vi "RADI SINHRO Peak Senzora.vi"() -> ()   [LabVIEW 2017]
uses:
  <vilib>/Waveform/WDTOps.llb/WDT Index Channel DBL.vi
panel:
  in  "Tab Control":enum32{"FRONT", "LIVE DATA", "Podesavanja"}(tab)
  in  "Brzina App":i16(slide)=1900 caption="Speed" min=500 max=1900 step=100 scale=500.0..1900.0
  out "3":bool
  out "2":bool
  out "1":bool
  out "?":dbl format="%#5_3g"
  out "TRENUTNI SIGNALI":dynamicdata(graph) caption="TRENUTNI SIGNALI !!!!"
  out "GORE":bool
  in  "Ponavljanja":i32=40
  out "ULAZ ANN":dbl[](array[numeric])
  out "Niz":dbl[](array[numeric])
  out "Matrica":dbl[][](array[numeric])
  out "BROJ":dbl
  out "SREDINA":bool
  out "DOLE":bool
  out "sum":dbl
  out "Sekvenca":dbl[](array[numeric])
  in  "Kombinacije":string(combo)="Combinations_1 - Srpski_Brojevi"
  out "Iter":i32
  out "SCORE":dbl
  in  "VREME 100mS":i16(knob)=1900 min=500 max=19000 step=100 scale=500.0..1900.0
  out "error out":errorcluster
  # "PROVERITI DA LI BROJ UDARCE"
  # "'Gore 1, Sredina 2, Dole 4, Miruje 8'"
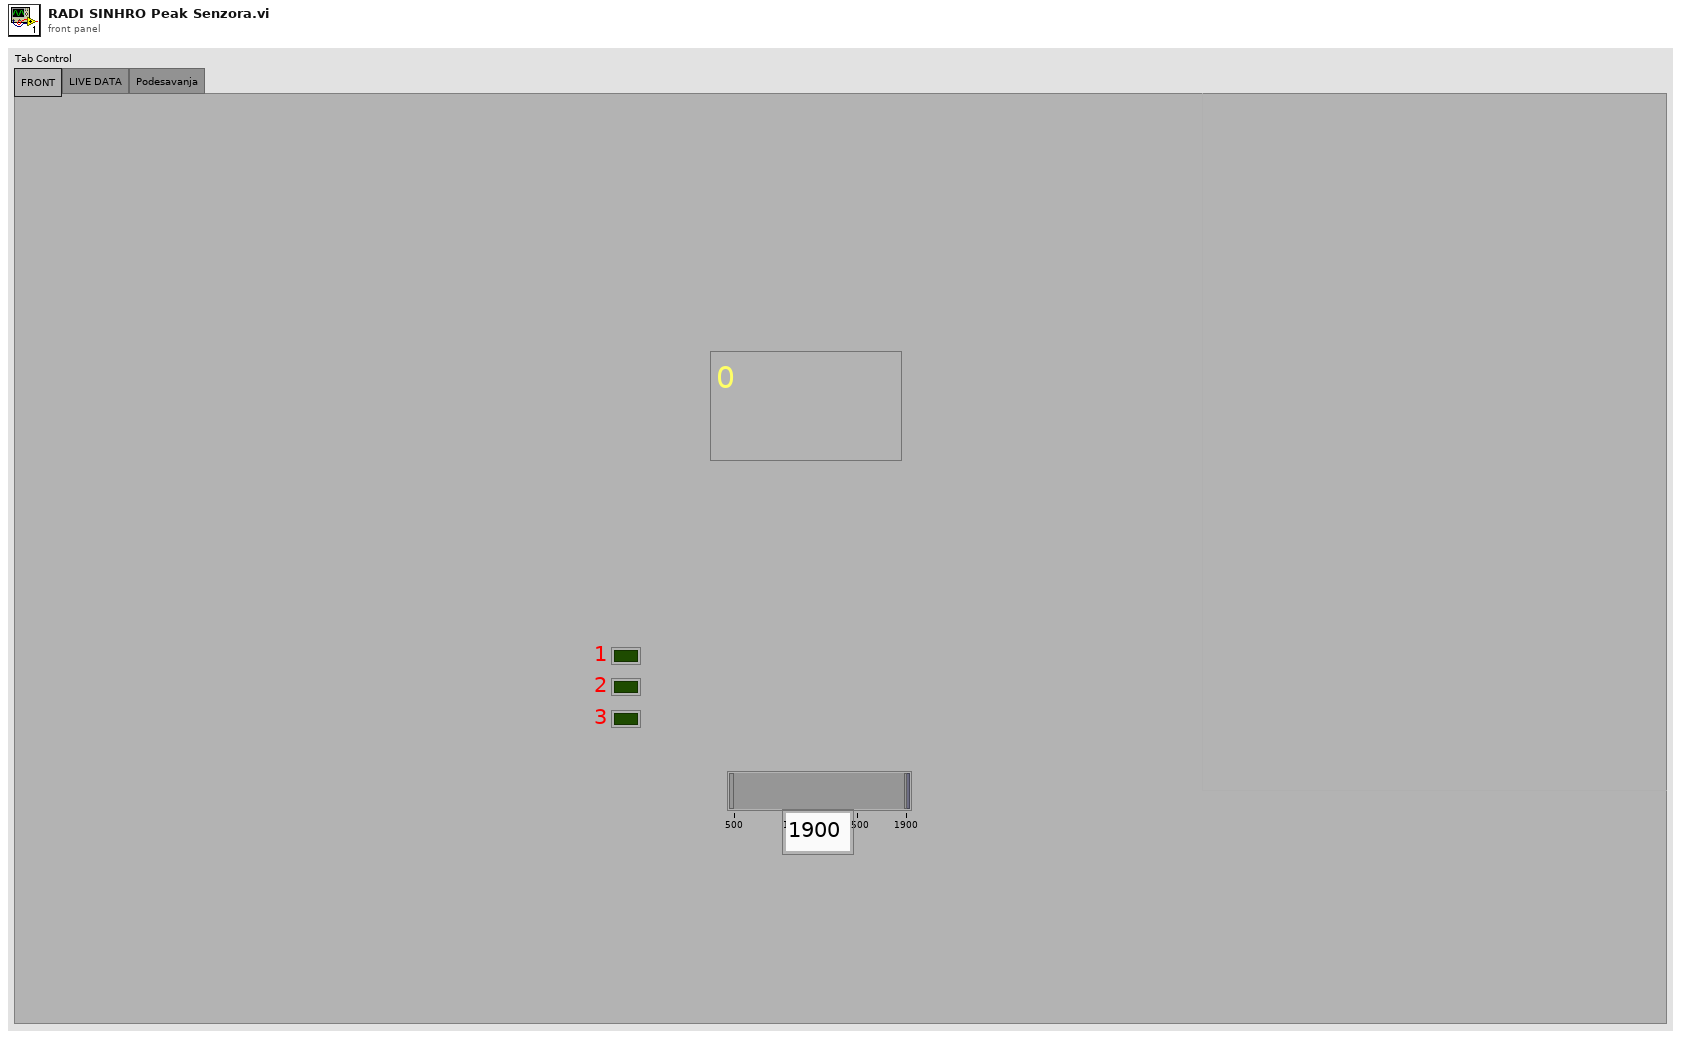
[diagram p1: front panel]
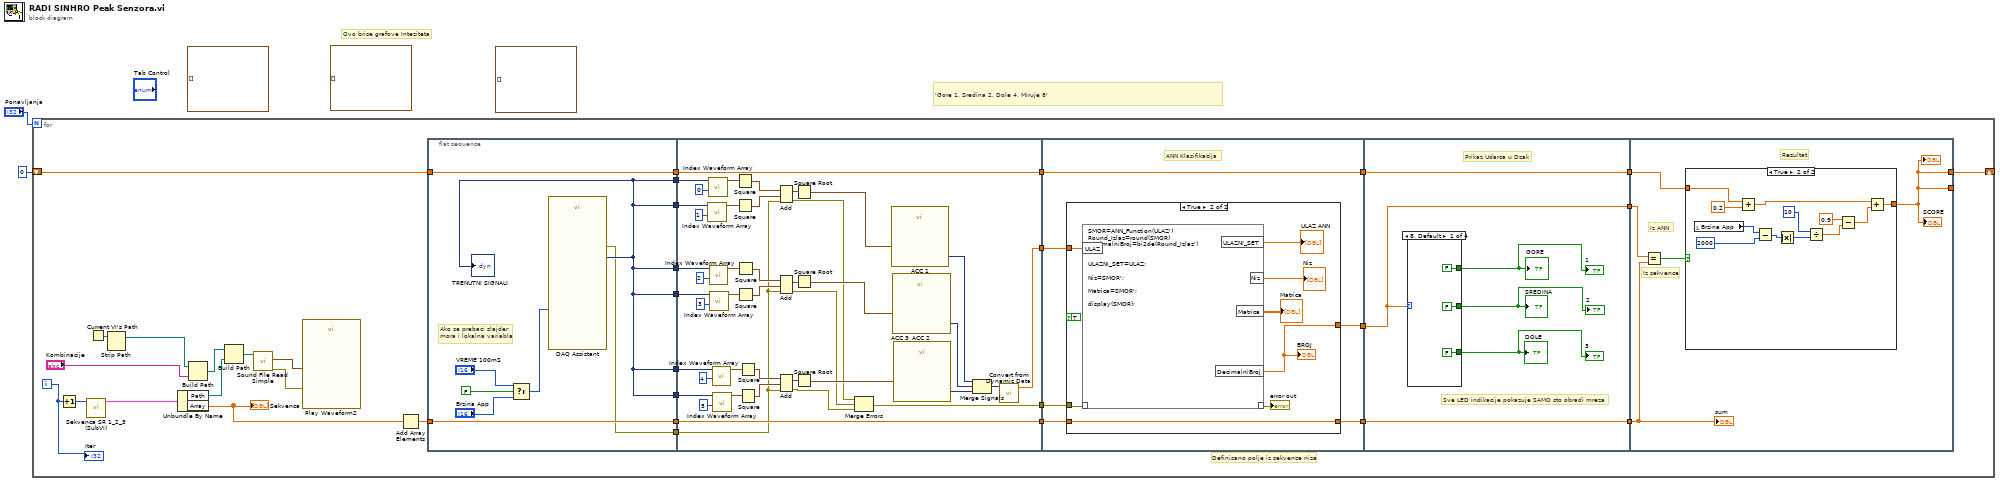
[diagram p0: block diagram]
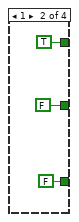
[diagram p3: hidden frame]
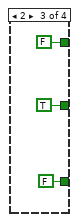
[diagram p4: hidden frame]
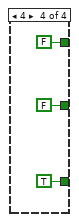
[diagram p5: hidden frame]
diagram:
  (unwired) waveform(dbl)[] [] ("History Data")
  (unwired) waveform(dbl)[] [] ("History Data")
  (unwired) waveform(dbl)[] [] ("History Data")
  # "'Gore 1, Sredina 2, Dole 4, Miruje 8'"
  # "Ovo brise grafove Inteziteta"
  n1 = for {
    N: "Ponavljanja" -> [_]
    shift-right: [w3] -> _
    shift-left: 0 -> [w25]
    i -> [w27]
    # "Definisano polje iz sekvence niza"
    n2 = Increment(x=w27) -> (x+1=w28:i32)
    n3 = call "Sekvenca SR 1_2_3 (SubVI).vi"("Ulaz"=w28) -> ("Cluster 41"=w29:cluster{"Path":path, "Array":dbl[]})  [unwired: 9 in, 1 out]
    n4 = Current VI's Path() -> (path=w35:path)
    n5 = Strip Path(path=w35) -> (stripped path=w32:path)  [unwired: 1 out]
    n6 = Unbundle By Name(w29) -> ("Path"=w30:path, "Array"=w26:dbl[])
    "Sekvenca" <- w26
    n7 = Build Path(base path=w32, name or relative path="Kombinacije") -> (appended path=w34:path)
    n8 = Build Path(base path=w34, name or relative path=w30) -> (appended path=w33:path)
    n9 = call <vilib>:"Sound File Read Simple.vi"("path"=w33) -> ("error out"=w36:errorcluster, "data"=w31:waveform(dbl)[])  [unwired: 7 in, 2 out]
    n10 = call "Play Waveform2"("Data"=w31, "error in"=w36) -> ()  [unwired: 17 in, 1 out]
    n11 = Add Array Elements(numeric array=w26) -> (sum=w19:dbl)
    n12 = flat-sequence {
      tunnel: w19 -> [w43]
      tunnel: w25 -> [w44]
      tunnel: [w44] -> w12
      tunnel: [w43] -> w11
      tunnel: [w41] -> w10
      tunnel: [w41] -> w9
      tunnel: [w41] -> w8
      tunnel: [w41] -> w7
      tunnel: [w41] -> w6
      tunnel: [w41] -> w5
      tunnel: [w37] -> w4
      tunnel: [w86] -> w16
      tunnel: [w47] -> w15
      tunnel: [w48] -> w14
      tunnel: [w85] -> w13
      tunnel: w12 -> [w86]
      tunnel: w11 -> [w85]
      tunnel: w10 -> [w59]
      tunnel: w9 -> [w57]
      tunnel: w8 -> [w55]
      tunnel: w7 -> [w53]
      tunnel: w6 -> [w51]
      tunnel: w5 -> [w49]
      tunnel: w4 -> [w45]
      tunnel: [w93] -> w21
      tunnel: [w87] -> w20
      tunnel: [w88] -> w17
      tunnel: w16 -> [w93]
      tunnel: w15 -> [w92]
      tunnel: w14 -> [w91]
      tunnel: w13 -> [w89]
      tunnel: [w105] -> w23
      tunnel: [w104] -> w22
      tunnel: w21 -> [w105]
      tunnel: w20 -> [w104]
      tunnel: [w103] -> w18
      tunnel: w17 -> [w103]
      tunnel: w23 -> [w124]
      tunnel: w22 -> [w122]
      tunnel: [w123] -> _
      tunnel: w18 -> [w121]
      tunnel: [w123] -> w3
      frame #0 {
        # "Ako se prebaci slajder\nmora i lokalna variabla"
        n13 = Select(t="VREME 100mS", s=FALSE, f="Brzina App") -> (s? t:f=w42:i16)
        n14 = call "DAQ Assistant"("number of samples"=w42) -> ("data"=w41:dynamicdata, "error out"=w37:errorcluster)  [unwired: 15 in, 2 out]
        "TRENUTNI SIGNALI" <- w41
      }
      frame #1 {
        n15 = call-poly <vilib>:"Index Waveform Array.vi"("index"=1, "waveform array"=w51) -> ("waveform"=w62:waveform(dbl))  [unwired: 8 in, 1 out]
        n16 = call-poly <vilib>:"Index Waveform Array.vi"("index"=0, "waveform array"=w49) -> ("waveform"=w61:waveform(dbl))  [unwired: 8 in, 1 out]
        n17 = call-poly <vilib>:"Index Waveform Array.vi"("index"=2, "waveform array"=w53) -> ("waveform"=w63:waveform(dbl))  [unwired: 8 in, 1 out]
        n18 = call-poly <vilib>:"Index Waveform Array.vi"("index"=3, "waveform array"=w55) -> ("waveform"=w64:waveform(dbl))  [unwired: 8 in, 1 out]
        n19 = call-poly <vilib>:"Index Waveform Array.vi"("index"=4, "waveform array"=w57) -> ("waveform"=w65:waveform(dbl))  [unwired: 8 in, 1 out]
        n20 = call-poly <vilib>:"Index Waveform Array.vi"("index"=5, "waveform array"=w59) -> ("waveform"=w66:waveform(dbl))  [unwired: 8 in, 1 out]
        n21 = Square(x=w61) -> (x^2=w67:waveform(dbl))
        n22 = Square(x=w62) -> (x^2=w68:waveform(dbl))
        n23 = Square(x=w63) -> (x^2=w69:waveform(dbl))
        n24 = Square(x=w64) -> (x^2=w70:waveform(dbl))
        n25 = Square(x=w65) -> (x^2=w71:waveform(dbl))
        n26 = Square(x=w66) -> (x^2=w72:waveform(dbl))
        n27 = Add(1:w68, 2:w67, 4:w45) -> (0:w73:waveform(dbl), 3:w76:errorcluster)
        n28 = Add(1:w70, 2:w69, 4:w45) -> (0:w74:waveform(dbl), 3:w77:errorcluster)
        n29 = Add(1:w72, 2:w71, 4:w45) -> (0:w75:waveform(dbl), 3:w78:errorcluster)
        n30 = Square Root(x=w73) -> (sqrt(x)=w81:waveform(dbl))
        n31 = Square Root(x=w74) -> (sqrt(x)=w82:waveform(dbl))
        n32 = Square Root(x=w75) -> (sqrt(x)=w83:waveform(dbl))
        n33 = Merge Errors(w76, w77, w78) -> (w47:errorcluster)
        n34 = call "ACC 1"("Signals"=w81) -> ("Peak to Peak"=w84:dynamicdata)  [unwired: 13 in, 1 out]
        n35 = call "ACC 2"("Signals"=w82) -> ("Peak to Peak"=w79:dynamicdata)  [unwired: 13 in, 1 out]
        n36 = call "ACC 3"("Signals"=w83) -> ("Peak to Peak"=w80:dynamicdata)  [unwired: 13 in, 1 out]
        n37 = Merge Signals(w84, w79, w80) -> (w46:dynamicdata)
        n38 = call "Convert from Dynamic Data"("Dynamic Data Type"=w46) -> ("Array"=w48:dbl[])  [unwired: 3 in]
      }
      frame #2 {
        # "ANN Klasifikacija"
        n39 = case shown="True" TRUE {
          tunnel: w92 -> [_ w102]
          tunnel: w91 -> [_ w101]
          tunnel: [_ w97] -> w87
          tunnel: [w94 w96] -> w88
          tunnel: w89 -> [w94 w96]
          frame False {
          }
          frame True {
            n40 = script code="SMOR=ANN_Function(ULAZ')\nRound_Izlaz=round(SMOR)\nDecimalniBroj=bi2de(Round_Izlaz')\n\n\nULAZNI_SET=ULAZ;\n\nNiz=SMOR';\n\nMatrica=SMOR';\n\ndisplay(SMOR);"("??"=w102, "ULAZ"=w101) -> ("??"=→"error out":errorcluster, "ULAZNI_SET"=→"ULAZ ANN":dbl[], "Niz"=→"Niz":dbl[], "Matrica"=→"Matrica":dbl[][], "DecimalniBroj"=w97:dbl)
            "BROJ" <- w97
          }
        }
      }
      frame #3 {
        # "Prikaz Udarca u Dzak"
        # "Sve LED indikacije pokazuje SAMO sto obradi mreza"
        n41 = case shown="8, Default" w104 {
          tunnel: [FALSE ("DOLE") FALSE ("DOLE") FALSE ("DOLE") TRUE ("DOLE")] -> w106
          tunnel: [FALSE ("SREDINA") FALSE ("SREDINA") TRUE ("SREDINA") FALSE ("SREDINA")] -> w107
          tunnel: [FALSE ("GORE") TRUE ("GORE") FALSE ("GORE") FALSE ("GORE")] -> w108
          frame 8, Default {
          }
          frame 1 {
          }
          frame 2 {
          }
          frame 4 {
          }
        }
        "GORE" <- w108
        "SREDINA" <- w107
        "DOLE" <- w106
        "1" <- w108
        "2" <- w107
        "3" <- w106
      }
      frame #4 {
        # "Rezultat"
        # "Iz sekvence"
        # "Iz ANN"
        n42 = Equal?(x=w122, y=w121) -> (x = y?=w125:bool)
        n43 = case shown="True" w125 {
          tunnel: w124 -> [w126 w128]
          tunnel: [w126 w127] -> w123
          frame False {
          }
          frame True {
            n44 = local read "Brzina App"() -> (w136:i16)
            n45 = Add(x=w128, y=0.2) -> (x+y=w133:dbl)
            n46 = Subtract(x=w136, y=2000) -> (x-y=w138:i32)
            n47 = Absolute Value(x=w138) -> (abs(x)=w137:i32)
            n48 = Divide(x=10, y=w137) -> (x/y=w135:dbl)
            n49 = Subtract(x=0.9, y=w135) -> (x-y=w134:dbl)
            n50 = Add(x=w133, y=w134) -> (x+y=w127:dbl)
          }
        }
        "SCORE" <- w123
        "?" <- w123
        "sum" <- w121
      }
    }
    "Iter" <- w27
  }
